vi "Move Splitters.vi"(4 "Old Width":i16, 6 "New Width":i16, 8 "error in":errorcluster, 10 "Left Splitter":refnum<vi>, 11 "Right Splitter":refnum<vi>) -> (0 "error out":errorcluster)   [LabVIEW 2023]
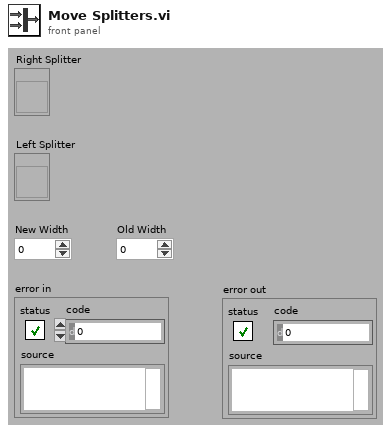
[diagram p1: front panel]
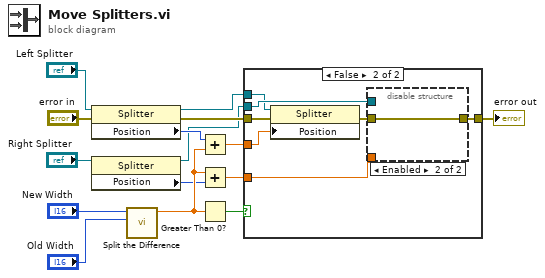
[diagram p0: block diagram]
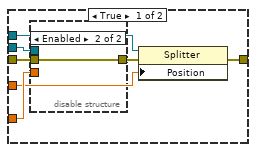
[diagram p2: hidden frame]
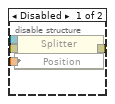
[diagram p3: hidden frame]
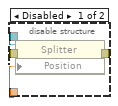
[diagram p4: hidden frame]
diagram:
  n1 = property class="Splitter"(reference="Left Splitter", error in="error in") -> (reference out=w8:refnum<vi>, error out=w5:errorcluster, "Position"=w10:i32)
  n2 = property class="Splitter"(reference="Right Splitter") -> (reference out=w1:refnum<vi>, "Position"=w2:i32)  [unwired: 1 in, 1 out]
  n3 = call "Split the Difference.vi"("Y"="Old Width", "X"="New Width") -> ("Half the Difference"=w3:dbl)  [unwired: 9 in]
  n4 = Add(x=w10, y=w3) -> (x+y=w11:dbl)
  n5 = Add(x=w3, y=w2) -> (x+y=w7:dbl)
  n6 = Greater Than 0?(x=w3) -> (x > 0?=w12:bool)
  n7 = case shown="False" w12 {
    tunnel: w5 -> [w22 w30]
    tunnel: w1 -> [w21 w34]
    tunnel: w7 -> [w20 w33]
    tunnel: w8 -> [w19 w32]
    tunnel: w11 -> [w18 w31]
    tunnel: [w16 w28] -> w13
    frame True {
      n8 = disable-structure shown="Enabled" {
        disable-tunnel: w22 -> [w26 w27]
        disable-tunnel: w21 -> [w25 _]
        disable-tunnel: w20 -> [w24 _]
        disable-tunnel: [w23 w27] -> w17
        frame Disabled {
          n9 = property class="Splitter"(reference=w25, error in=w26, "Position"=w24) -> (error out=w23:errorcluster)  [unwired: 1 out]
        }
        frame Enabled {
        }
      }
      n10 = property class="Splitter"(reference=w19, error in=w17, "Position"=w18) -> (error out=w16:errorcluster)  [unwired: 1 out]
    }
    frame False {
      n11 = property class="Splitter"(reference=w32, error in=w30, "Position"=w31) -> (error out=w29:errorcluster)  [unwired: 1 out]
      n12 = disable-structure shown="Enabled" {
        disable-tunnel: w34 -> [w38 _]
        disable-tunnel: w33 -> [w37 _]
        disable-tunnel: w29 -> [w36 w39]
        disable-tunnel: [w35 w39] -> w28
        frame Disabled {
          n13 = property class="Splitter"(reference=w38, error in=w36, "Position"=w37) -> (error out=w35:errorcluster)  [unwired: 1 out]
        }
        frame Enabled {
        }
      }
    }
  }
  "error out" <- w13
